vi "Tektronix 7000 Series Read Waveform From File.vi"() -> ()   [LabVIEW 2015]
doc: "This example VI illustrates how to Read data from File using the following steps. This VI will read less than 100000 points from the file. \n1. Specify a Path where you save the waveform data.\n2. Set Start and End Position.\n3. Run the VI and Get the Measurement.\n\n<B>Note:</B> The data displayed in the graph will be decimated. See the block diagram for more details."
uses:
  <instrlib>/Tektronix 7000 Series/Tektronix 7000 Series.lvlib
panel:
  out "Waveform Graph":waveform(sgl)(graph)
  out "Start Time":sgl
  out "Count":i32
  out "Time Interval":sgl
  in  "Filename (C:\\data.txt)":path=path "C:/data.txt"
  in  "End Position (100%)":dbl=100.0
  in  "Start Position (0%)":dbl
  # "(c) 2006 - 2016 National Instruments Corporation.  ALL RIGHTS RESERVED."
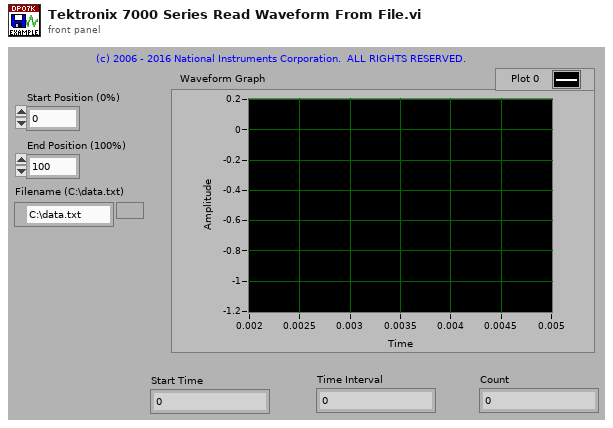
[diagram p1: front panel]
types:
  T1 = enum16{"open", "open or create", "create or replace", "create", "open (read only)"}
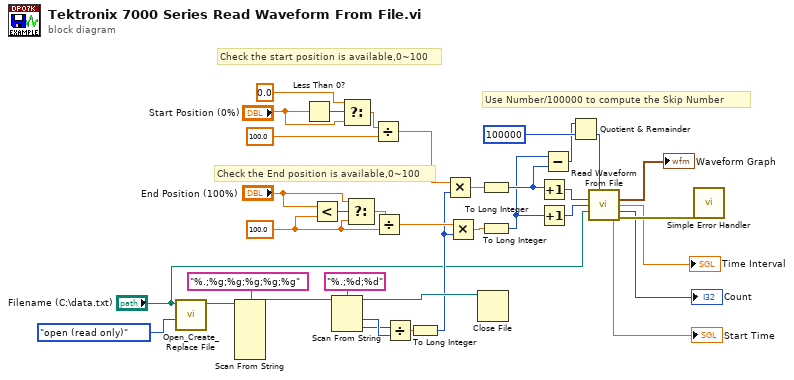
[diagram p0: block diagram]
diagram:
  w18 = 100.0 ("y")
  # "Use Number/100000 to compute the Skip Number"
  # "Check the End position is available,0~100"
  # "Check the start position is available,0~100"
  n1 = call <vilib>:"Open_Create_Replace File.vi"("function (open:0)"=T1."open (read only)", "file path"="Filename (C:\\data.txt)") -> ("refnum"=w33:refnum<file>)  [unwired: 6 in, 3 out]
  n2 = Scan From String("%.;%g;%g;%g;%g;%g" ("format string"), w33) -> (w32:refnum<file>)  [unwired: 11 in, 1 out]
  n3 = Less Than 0?(x="Start Position (0%)") -> (x < 0?=w25:bool)
  n4 = Less?(x="End Position (100%)", y=w18) -> (x < y?=w19:bool)
  n5 = Scan From String("%.;%d;%d" ("format string"), w32) -> (w27:refnum<file>, output 1=w29:i32, output 2=w28:i32)  [unwired: 3 in, 1 out]
  n6 = Select(t=0.0, s=w25, f="Start Position (0%)") -> (s? t:f=w23:dbl)
  n7 = Select(t="End Position (100%)", s=w19, f=w18) -> (s? t:f=w17:dbl)
  n8 = Divide(x=w23, y=100.0) -> (x/y=w20:dbl)
  n9 = Divide(x=w17, y=w18) -> (x/y=w15:dbl)
  n10 = Divide(x=w28, y=w29) -> (x/y=w30:dbl)
  n11 = To Long Integer(number=w30) -> (32bit integer=w14:i32)
  n12 = Multiply(x=w20, y=w14) -> (x*y=w26:dbl)
  n13 = Multiply(x=w15, y=w14) -> (x*y=w13:dbl)
  n14 = Close File(refnum=w27) -> ()  [unwired: 1 in, 2 out]
  n15 = To Long Integer(number=w26) -> (32bit integer=w8:i32)
  n16 = To Long Integer(number=w13) -> (32bit integer=w6:i32)
  n17 = Increment(x=w8) -> (x+1=w7:i32)
  n18 = Increment(x=w6) -> (x+1=w5:i32)
  n19 = Subtract(x=w6, y=w8) -> (x-y=w11:i32)
  n20 = Quotient & Remainder(x=w11, y=100000) -> (floor(x/y)=w10:i32)  [unwired: 1 out]
  n21 = call <instrlib>:"Read Waveform From File.vi"("Skip N Points (1)"=w10, "Start Point (1)"=w7, "End Point (10000)"=w5, "Filename (C:\\data.txt)"="Filename (C:\\data.txt)") -> ("Waveform Graph"=→"Waveform Graph":waveform(sgl), "Time Interval"=→"Time Interval":sgl, "Count"=→"Count":i32, "Start Time"=→"Start Time":sgl, "error out"=w36:errorcluster)  [unwired: 6 in, 1 out]
  n22 = call <vilib>:"Simple Error Handler.vi"("error in (no error)"=w36) -> ()  [unwired: 4 in, 5 out]
